vi "GUI_Magspec_BELLA_Line.vi"() -> ()   [LabVIEW 2013]
uses:
  shared programs/GUI_Template/GUI_master/tcp_new_data_event.ctl
  shared programs/GUI_Template/GUI_master/tcp new data cluster.ctl
  <vilib>/Analysis/2dsp.llb/Decimate (single shot, DBL).vi
  <vilib>/Analysis/NI_AALPro.lvlib
panel:
  in  "rank for LPF":i32=2
  out "Momentum 25":dbl=2.780793 caption="Momentum (GeV/c)" min=0.0 max=0.0 format="%#.1f"
  out "Momentum 24":dbl=2.780793 caption="Momentum (GeV/c)" min=0.0 max=0.0 format="%#.1f"
  out "Momentum 23":dbl=2.780793 caption="Momentum (GeV/c)" min=0.0 max=0.0 format="%#.1f"
  out "Momentum 22":dbl=2.780793 caption="Momentum (GeV/c)" min=0.0 max=0.0 format="%#.1f"
  out "Momentum 21":dbl=2.780793 caption="Momentum (GeV/c)" min=0.0 max=0.0 format="%#.1f"
  out "Momentum 20":dbl=2.780793 caption="Momentum (GeV/c)" min=0.0 max=0.0 format="%#.1f"
  out "Momentum 19":dbl=2.780793 caption="Momentum (GeV/c)" min=0.0 max=0.0 format="%#.1f"
  out "Momentum 18":dbl=2.780793 caption="Momentum (GeV/c)" min=0.0 max=0.0 format="%#.1f"
  out "Momentum 17":dbl=2.780793 caption="Momentum (GeV/c)" min=0.0 max=0.0 format="%#.1f"
  out "Momentum 16":dbl=2.780793 caption="Momentum (GeV/c)" min=0.0 max=0.0 format="%#.1f"
  out "Momentum 15":dbl=2.780793 caption="Momentum (GeV/c)" min=0.0 max=0.0 format="%#.1f"
  out "Waveform Graph":dbl[](graph)
  in  "HorizontalLineout::12":dbl[](array[numeric]) caption="HorizontalLineout MagSpecA"
  in  "HorizontalLineout::11":dbl[](array[numeric]) caption="HorizontalLineout MagSpecA"
  in  "HorizontalLineout::10":dbl[](array[numeric]) caption="HorizontalLineout MagSpecA"
  in  "HorizontalLineout::9":dbl[](array[numeric]) caption="HorizontalLineout MagSpecA"
  in  "HorizontalLineout::8":dbl[](array[numeric]) caption="HorizontalLineout MagSpecA"
  in  "HorizontalLineout::7":dbl[](array[numeric]) caption="HorizontalLineout MagSpecA"
  in  "HorizontalLineout::6":dbl[](array[numeric]) caption="HorizontalLineout MagSpecA"
  in  "HorizontalLineout::5":dbl[](array[numeric]) caption="HorizontalLineout MagSpecA"
  in  "HorizontalLineout::4":dbl[](array[numeric]) caption="HorizontalLineout MagSpecA"
  in  "HorizontalLineout::3":dbl[](array[numeric]) caption="HorizontalLineout MagSpecA"
  in  "HorizontalLineout::2":dbl[](array[numeric]) caption="HorizontalLineout MagSpecA"
  in  "HorizontalLineout::1":dbl[](array[numeric]) caption="HorizontalLineout MagSpecA"
  in  "GUIdevice 14":string="BELLA_HallProbe"
  in  "GUIdevice 12":string="MagSpecL"
  in  "GUIdevice 11":string="MagSpecK"
  in  "GUIdevice 10":string="MagSpecJ"
  in  "GUIdevice 9":string="MagSpecI"
  in  "GUIdevice 8":string="MagSpecH"
  in  "GUIdevice 7":string="MagSpecG"
  in  "GUIdevice 6":string="MagSpecF"
  in  "GUIdevice 5":string="MagSpecE"
  in  "GUIdevice 4":string="MagSpecD"
  in  "GUIdevice 3":string="MagSpecC"
  in  "GUIdevice 2":string="MagSpecB"
  in  "Field::14":dbl=2.780793 caption="Magnetic Field (mT)" min=0.0 max=0.0 format="%_4f"
  in  "GUIdevice 13":string="EBeam_Profile_BELLA_1"
  in  "GUIdevice 1":string="MagSpecA"
  out "tcp data event":T1
  in  "stop":bool
  out "error IO 2":errorcluster
  out "Boolean":bool
  # "MeV/c"
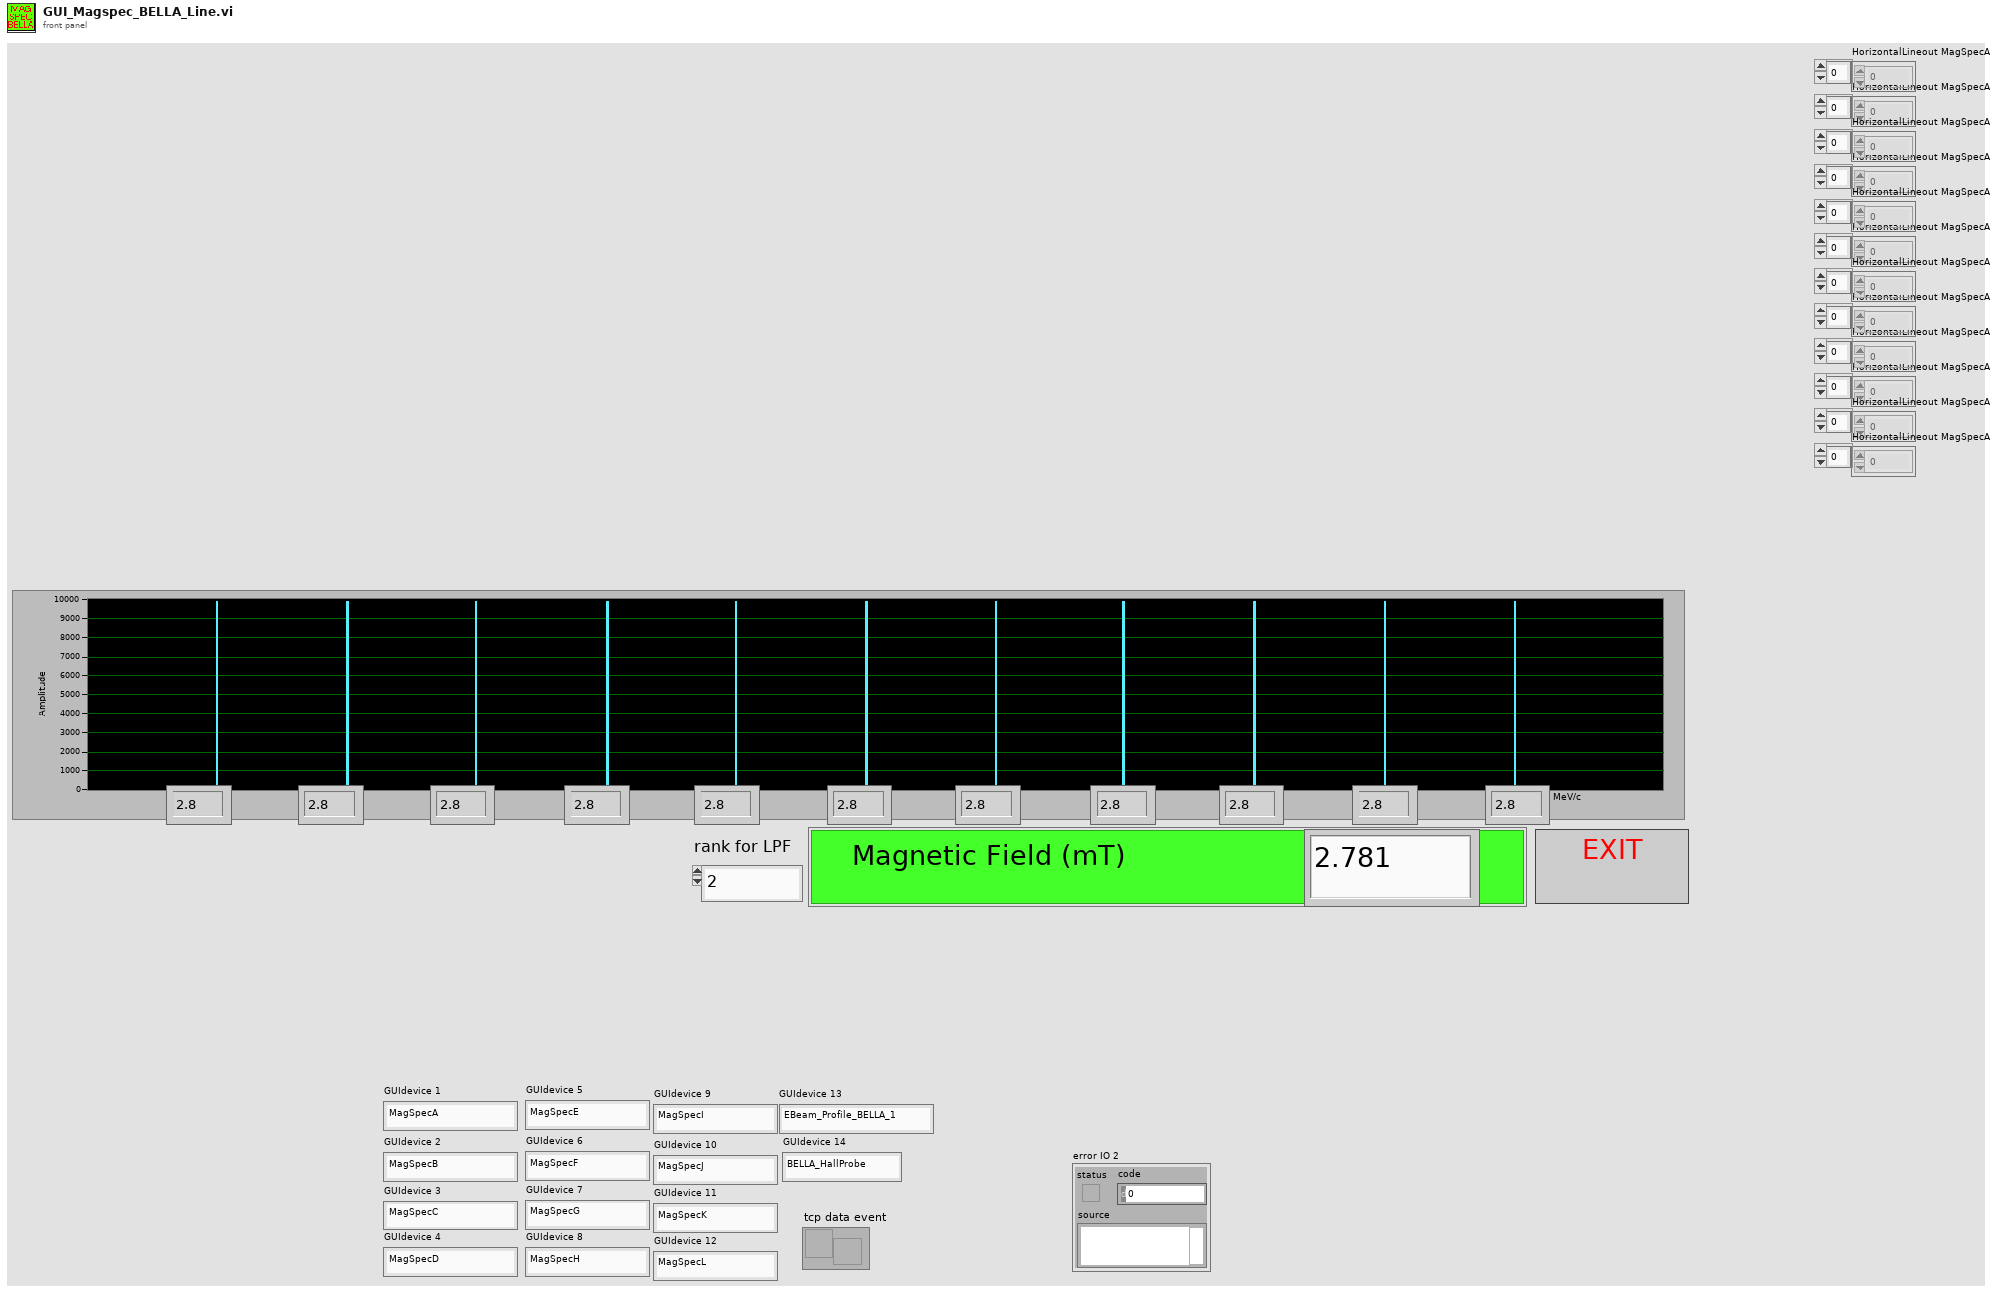
[diagram p1: front panel]
types:
  T1 = typedef "tcp_new_data_event.ctl" = refnum<user-event>
  T2 = typedef "tcp new data cluster.ctl" = cluster{"EventEnum":enum16{"new data", "connection status update"}, "Device name":string}
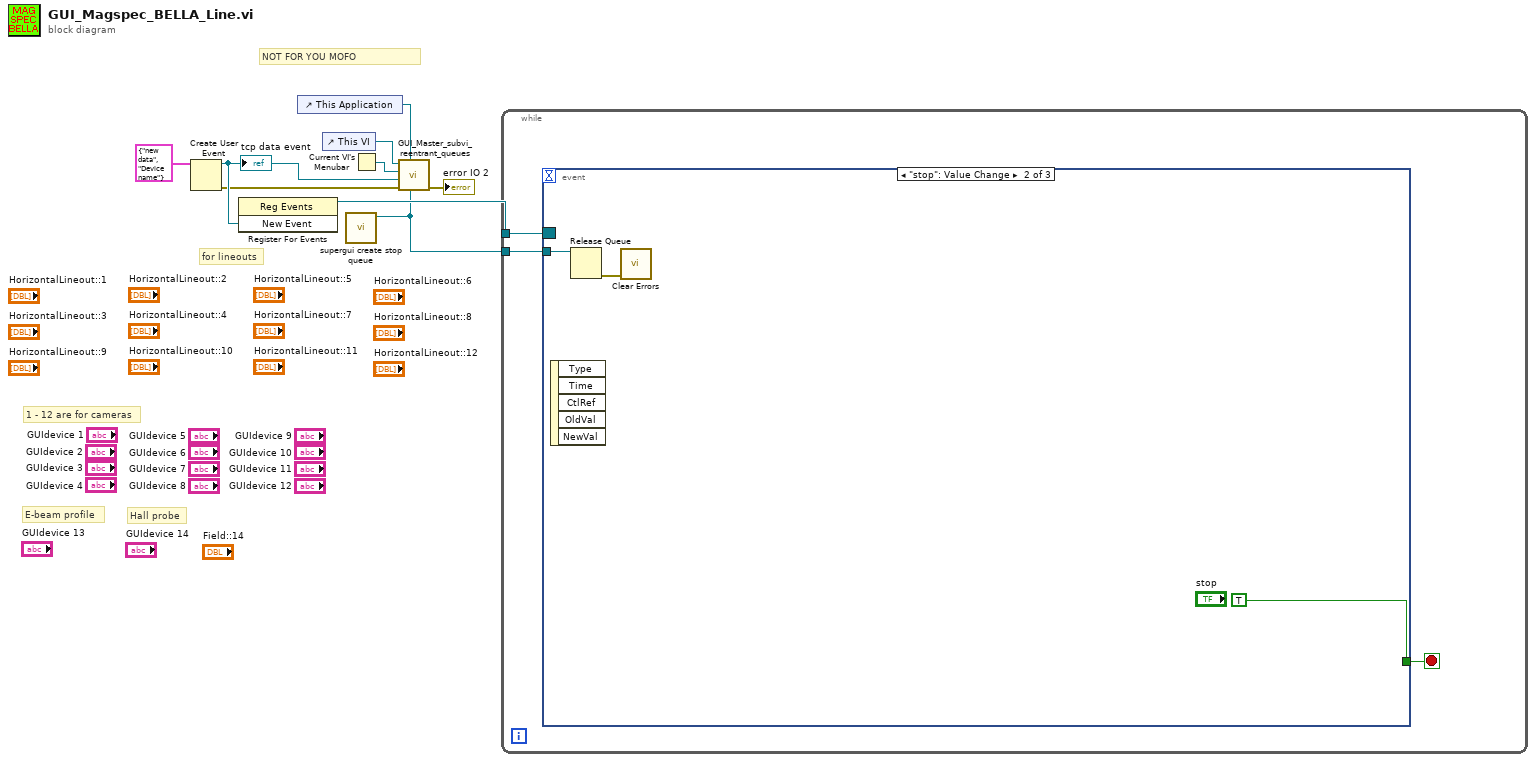
[diagram p0: block diagram]
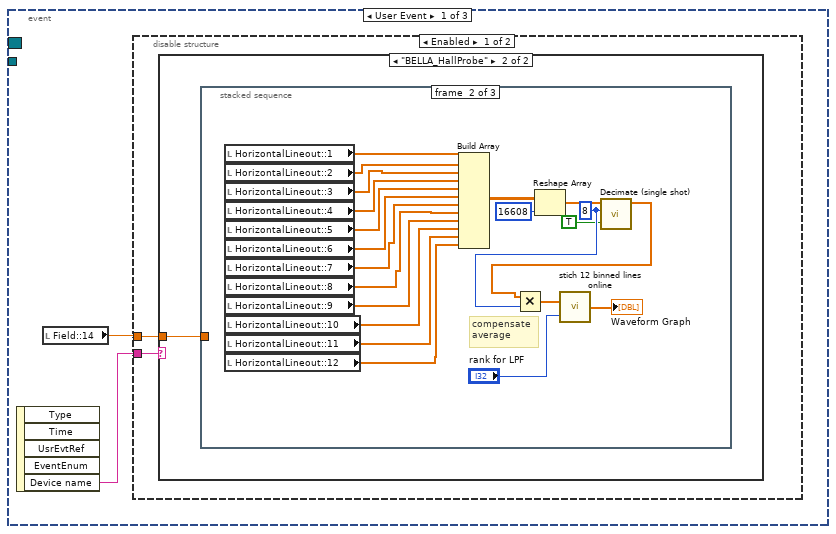
[diagram p2: hidden frame]
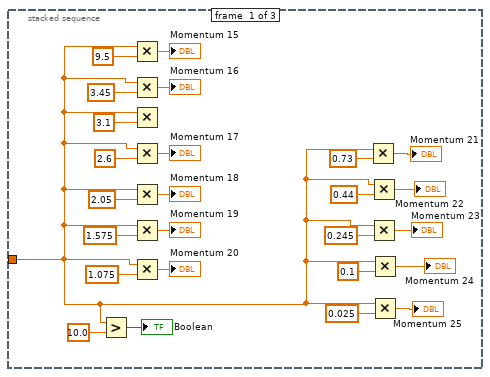
[diagram p4: hidden frame]
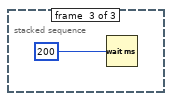
[diagram p5: hidden frame]
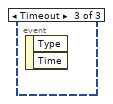
[diagram p7: hidden frame]
diagram:
  # "for lineouts"
  # "Hall probe"
  # "E-beam profile"
  # "1 - 12 are for cameras"
  # "NOT FOR YOU MOFO"
  n1 = Create User Event(user event datatype=T2 {"EventEnum"=enum."new data", "Device name"="Device name"} ("New Event")) -> (user event=w8:refnum<user-event>, error out=w7:errorcluster)  [unwired: 1 in]
  "tcp data event" <- w8
  n2 = register-events(w8) -> (reference out=w3:refnum<event-registration>)  [unwired: 2 in, 1 out]
  n3 = control-ref of="This Application"() -> (w9:refnum<vi>)
  n4 = control-ref of="This VI"() -> (w4:refnum<vi>)
  n5 = call "supergui create stop queue.vi"() -> ("STOP Queue out"=w1:refnum<queue>)  [unwired: 11 in]
  n6 = Current VI's Menubar() -> (w5:refnum<k9>)
  n7 = call "GUI_Master_subvi_reentrant_queues.vi"("STOP Queue in"=w1, "This Application"=w9, "error in (no error)"=w7, "tcp data event"=w8, "Caller menu reference"=w5, "Caller VI ref"=w4) -> ("error out"=→"error IO 2":errorcluster)  [unwired: 5 in]
  n8 = while {
    tunnel: w3 -> [w11]
    tunnel: w1 -> [w10]
    stop <- w12 stop-if-true
    n9 = event shown="[1] \"stop\": Value Change" {
      selector: w11 -> [_ _ _]
      dyn-events: _ -> [_ _ _]
      timeout: _ -> [_ _ _]
      tunnel: [_ TRUE ("stop") _] -> w12
      tunnel: w10 -> [_ w67 _]
      event User Event {
        n10 = event-data() -> ("Device name"=w14:string)  [unwired: 1 in, 4 out]
        n11 = local read "Field::14"() -> (w13:dbl)
        n12 = disable-structure shown="Enabled" {
          disable-tunnel: w14 -> [w16 _]
          disable-tunnel: w13 -> [w15 _]
          frame Enabled {
            n13 = case shown="\"BELLA_HallProbe\"" w16 {
              tunnel: w15 -> [_ w17]
              frame "False", Default {
              }
              frame "BELLA_HallProbe" {
                n14 = stacked-sequence {
                  tunnel: w17 -> [w18 _ _]
                  frame #0 {
                    n15 = Greater?(x=w18, y=10.0) -> (0:→"Boolean":bool)
                    n16 = Multiply(x=w18, y=9.5) -> (x*y=→"Momentum 15":dbl)
                    n17 = Multiply(x=w18, y=3.45) -> (x*y=→"Momentum 16":dbl)
                    n18 = Multiply(x=w18, y=3.1) -> ()  [unwired: 1 out]
                    n19 = Multiply(x=w18, y=2.6) -> (x*y=→"Momentum 17":dbl)
                    n20 = Multiply(x=w18, y=2.05) -> (x*y=→"Momentum 18":dbl)
                    n21 = Multiply(x=w18, y=1.575) -> (x*y=→"Momentum 19":dbl)
                    n22 = Multiply(x=w18, y=1.075) -> (x*y=→"Momentum 20":dbl)
                    n23 = Multiply(x=w18, y=0.73) -> (x*y=→"Momentum 21":dbl)
                    n24 = Multiply(x=w18, y=0.44) -> (x*y=→"Momentum 22":dbl)
                    n25 = Multiply(x=w18, y=0.245) -> (x*y=→"Momentum 23":dbl)
                    n26 = Multiply(x=w18, y=0.1) -> (x*y=→"Momentum 24":dbl)
                    n27 = Multiply(x=w18, y=0.025) -> (x*y=→"Momentum 25":dbl)
                  }
                  frame #1 {
                    w63 = 8 ("decimating factor")
                    # "compensate\naverage"
                    n28 = local read "HorizontalLineout::1"() -> (w44:dbl[])
                    n29 = local read "HorizontalLineout::2"() -> (w45:dbl[])
                    n30 = local read "HorizontalLineout::3"() -> (w46:dbl[])
                    n31 = local read "HorizontalLineout::4"() -> (w47:dbl[])
                    n32 = local read "HorizontalLineout::5"() -> (w48:dbl[])
                    n33 = local read "HorizontalLineout::6"() -> (w49:dbl[])
                    n34 = local read "HorizontalLineout::7"() -> (w50:dbl[])
                    n35 = local read "HorizontalLineout::8"() -> (w51:dbl[])
                    n36 = local read "HorizontalLineout::9"() -> (w52:dbl[])
                    n37 = local read "HorizontalLineout::10"() -> (w53:dbl[])
                    n38 = local read "HorizontalLineout::11"() -> (w54:dbl[])
                    n39 = local read "HorizontalLineout::12"() -> (w55:dbl[])
                    n40 = Build Array(w44, w45, w46, w47, w48, w49, w50, w51, w52, w53, w54, w55) -> (w56:dbl[][])
                    n41 = Reshape Array(w56, 16608 ("dimension size")) -> (w58:dbl[])
                    n42 = call-poly <vilib>:"Decimate (single shot).vi"("averaging"=TRUE, "decimating factor"=w63, "X"=w58) -> ("Decimated Array"=w62:dbl[])  [unwired: 7 in, 1 out]
                    n43 = Multiply(x=w62, y=w63) -> (x*y=w61:dbl[])
                    n44 = call "stich 12 binned lines online.vi"("rank"="rank for LPF", "Input"=w61) -> ("stiched signal"=→"Waveform Graph":dbl[])
                  }
                  frame #2 {
                    n45 = Wait (ms)(milliseconds to wait=u32 200 ("delay")) -> ()  [unwired: 1 out]
                  }
                }
              }
            }
          }
          frame Disabled {
          }
        }
      }
      event "stop": Value Change {
        n46 = event-data() -> ()  [unwired: 1 in, 5 out]
        n47 = Release Queue(queue=w67) -> (error out=w66:errorcluster)  [unwired: 2 in, 2 out]
        n48 = call <vilib>:"Clear Errors.vi"("error in (no error)"=w66) -> ()  [unwired: 6 in, 1 out]
      }
      event Timeout {
        n49 = event-data() -> ()  [unwired: 1 in, 2 out]
      }
    }
  }
